vi "LevMar - Target Caller.vi"(0 "A":dbl[](array[numeric]), 1 "Target Function in":refnum<vi>) -> (2 "Target Function out":refnum<vi>, 3 "F":dbl[](array[numeric]))   [LabVIEW 2009]
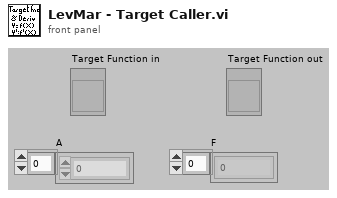
[diagram p1: front panel]
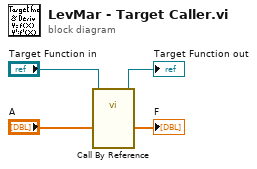
[diagram p0: block diagram]
diagram:
  n1 = call-by-ref "?"(reference="Target Function in", "A"="A") -> (reference out=→"Target Function out":refnum<vi>, "F"=→"F":dbl[])  [unwired: 1 in, 1 out]
